vi "Load Sample Custom VI.vi"(8 "error in":errorcluster, 10 "Title":string, 11 "Template":refnum<class "MetaDataObj.lvclass">) -> (0 "error out":errorcluster, 2 "Path":path, 3 "Template out":refnum<class "MetaDataObj.lvclass">)   [LabVIEW 2021]
uses:
  <resource>/dialog/NewProjectWizard/MetaDataObj/MetaDataObj.lvclass
  <resource>/dialog/NewProjectWizard/MetaDataObj/Accessors/Read LocationPath.vi
  <vilib>/xml/Load XML File.vi
  <vilib>/xml/Close Reference(Node).vi
  <resource>/dialog/NewProjectWizard/MetaDataObj/Accessors/Write Custom VI Path.vi
  <vilib>/myRIO/Common/FPGA Personality Framework/Personality.lvlib
  <vilib>/xml/NI_XML.lvlib
  <resource>/dialog/NewProjectWizard/Loading Project Info/NI_NPW_Loading Project Info.lvlib
  myRIOMetaDataObj/myRIOMetaDataObj.lvclass
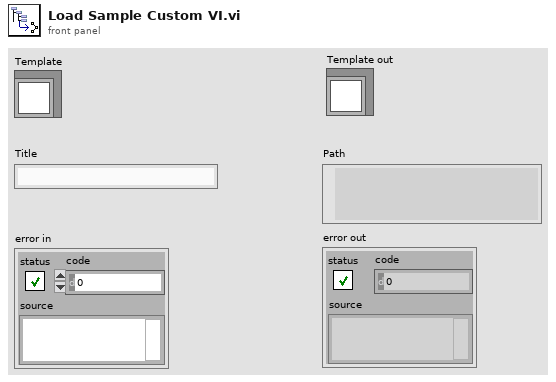
[diagram p1: front panel]
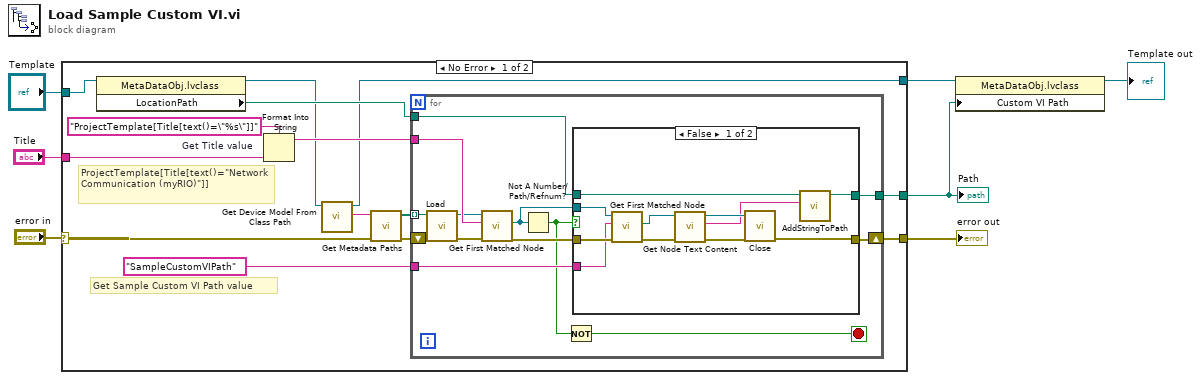
[diagram p0: block diagram]
diagram:
  n1 = case shown="No Error" "error in" {
    selector: "error in" -> [w21 w48]
    tunnel: "Title" -> [w18 _]
    tunnel: [w14 _] -> w2
    tunnel: [w13 w48] -> w5
    tunnel: "Template" -> [w12 w47]
    tunnel: [w8 w47] -> w3
    frame No Error {
      w17 = "ProjectTemplate[Title[text()=\"%s\"]]"  # Get Title value
      # "ProjectTemplate[Title[text()=\"Network Communication (myRIO)\"]]"
      # "Get Sample Custom VI Path value"
      n2 = property class="MetaDataObj.lvclass"(reference=w12) -> (reference out=w9:refnum<class "MetaDataObj.lvclass">, "LocationPath"=w11:path)  [unwired: 1 in, 1 out]
      n3 = Format Into String(format string=w17, w18) -> (resulting string=w16:string)  [unwired: 2 in, 1 out]
      n4 = call "Get Device Model From Class Path.vi"("MetaDataObj in"=w9) -> ("Device Model Str"=w10:string, "MetaDataObj Out"=w8:refnum<class "MetaDataObj.lvclass">)  [unwired: 8 in, 1 out]
      n5 = call <vilib>:"Get Metadata Paths.vi"("error in (no error)"=w21, "Device Model Str"=w10) -> ("error out"=w20:errorcluster, "Meta Data File Paths"=w19:path[])  [unwired: 8 in]
      n6 = for {
        tunnel: w19 -> [w33] mode=indexing
        shift-right: [w26] -> w13
        shift-left: w20 -> [w34]
        tunnel: w16 -> [w32]
        tunnel: "SampleCustomVIPath" -> [w28]
        tunnel: [w25] -> w14
        tunnel: w11 -> [w24]
        stop <- w22 stop-if-true
        n7 = call-poly <vilib>:"Load.vi"("path to XML document"=w33, "error in (no error)"=w34) -> ("DOM document out"=w31:refnum<k20>, "error out"=w30:errorcluster)  [unwired: 11 in, 1 out]
        n8 = call <vilib>:"Get First Matched Node.vi"("error in (no error)"=w30, "XPath expression"=w32, "node in"=w31) -> ("error out"=w29:errorcluster, "node result"=w27:refnum<k20>)  [unwired: 6 in, 1 out]
        n9 = Not A Number/Path/Refnum?(number/path/refnum=w27) -> (NaN/Path/Refnum?=w23:bool)
        n10 = Not(x=w23) -> (.not. x?=w22:bool)
        n11 = case shown="False" w23 {
          tunnel: w29 -> [w44 w46]
          tunnel: w28 -> [w43 _]
          tunnel: w27 -> [w42 _]
          tunnel: [w38 w46] -> w26
          tunnel: [w36 _] -> w25
          tunnel: w24 -> [w35 _]
          frame False {
            n12 = call <vilib>:"Get First Matched Node.vi"("error in (no error)"=w44, "XPath expression"=w43, "node in"=w42) -> ("error out"=w45:errorcluster, "node result"=w41:refnum<k20>)  [unwired: 6 in, 1 out]
            n13 = call <vilib>:"Get Node Text Content.vi"("error in (no error)"=w45, "node in"=w41) -> ("error out"=w40:errorcluster, "node text"=w37:string, "node out"=w39:refnum<k20>)  [unwired: 7 in]
            n14 = call-poly <vilib>:"Close.vi"("error in (no error)"=w40, "node"=w39) -> ("error out"=w38:errorcluster)  [unwired: 7 in]
            n15 = call <resource>:"AddStringToPath.vi"("String"=w37, "Path In"=w35) -> ("Path Out"=w36:path)  [unwired: 9 in]
          }
          frame True {
          }
        }
      }
    }
    frame Error {
    }
  }
  "error out" <- w5
  "Path" <- w2
  n16 = property class="MetaDataObj.lvclass"(reference=w3, "Custom VI Path"=w2) -> (reference out=→"Template out":refnum<class "MetaDataObj.lvclass">)  [unwired: 1 in, 1 out]
